vi "From JSON String.vi"(8 "error in (no error)":errorcluster, 10 "JSON String":string, 11 "JSONable in":refnum<class "JSONable.lvclass">) -> (0 "error out":errorcluster, 3 "JSONable out":refnum<class "JSONable.lvclass">)   [LabVIEW 2015, in "JSONable.lvclass"]
uses:
  JSONable.lvclass
  <vilib>/rajsite/i3-json/i3-json.lvlib
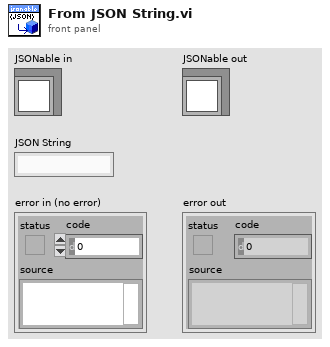
[diagram p1: front panel]
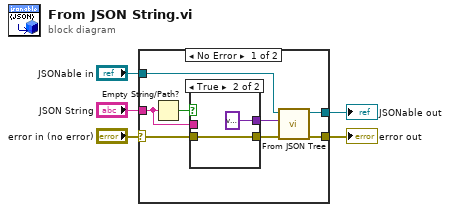
[diagram p0: block diagram]
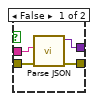
[diagram p2: hidden frame]
diagram:
  n1 = case shown="No Error" "error in (no error)" {
    selector: "error in (no error)" -> [w9 w21]
    tunnel: [w11 w21] -> w4
    tunnel: [w12 w20] -> w2
    tunnel: "JSONable in" -> [w13 w20]
    tunnel: "JSON String" -> [w7 _]
    frame No Error {
      n2 = Empty String/Path?(string/path=w7) -> (empty?=w6:bool)
      n3 = case shown="True" w6 {
        tunnel: w7 -> [w17 _]
        tunnel: [w16 variant ("JSON Tree")] -> w10
        tunnel: w9 -> [w15 w18]
        tunnel: [w14 w18] -> w8
        frame False {
          n4 = call <vilib>:"Parse JSON.vi"("error in (no error)"=w15, "JSON String"=w17) -> ("error out"=w14:errorcluster, "JSON Tree"=w16:variant)  [unwired: 6 in, 2 out]
        }
        frame True {
        }
      }
      n5 = call-dynamic "From JSON Tree.vi"("error in (no error)"=w8, "JSON Tree In"=w10, "JSONable in"=w13) -> ("error out"=w11:errorcluster, "JSONable out"=w12:refnum<class "JSONable.lvclass">)  [unwired: 7 in]
    }
    frame Error {
    }
  }
  "error out" <- w4
  "JSONable out" <- w2
